vi "N-216 Stage Engine.vi"(0 "Unique Notifier Name":string, 11 "COM Port":string[](array[string])) -> ()   [LabVIEW 2016]
uses:
  Stages Controls/Stage Focus Control.ctl
  Stages Controls/Stage Status.ctl
  Stages Controls/Stage Actions.ctl
  Stages Controls/Stage Notifier Element.ctl
  PI GCS2 DLL/PI_GCS2_DLL_x64.dll
panel:
  in  "Reference":bool
  in  "Velocity (µm/s)":dbl=0.1 format="%#_13g"
  out "Number Connected":i32
  out "E-712 Found":bool
  in  "ReInitialize":bool
  in  "Abort":bool
  out "Status":T1
  in  "QUIT":bool
  in  "Focus Control":T2
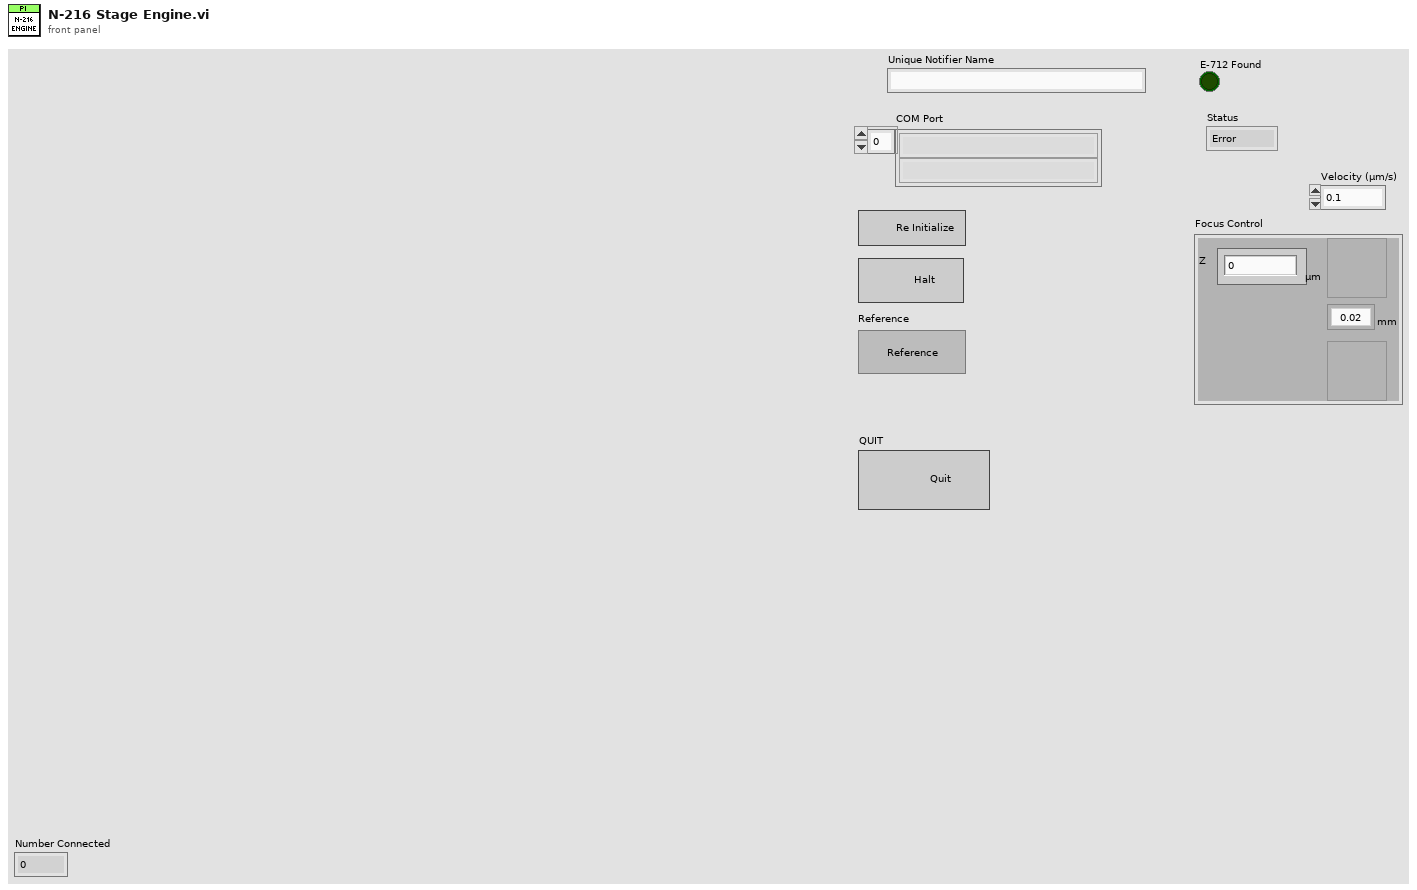
[diagram p1: front panel]
types:
  T1 = typedef "Stage Status.ctl" = enum16{"Error", "Abort", "Busy", "On Target"}
  T2 = typedef "Stage Focus Control.ctl" = cluster{"Focus Step (um)":enum16{"0.02", "0.05", "0.1", "0.5", "1", "2", "5", "10", "20"}, "Focus Up":bool, "Focus Down":bool, "Z ":dbl}
  T3 = typedef "Stage Notifier Element.ctl" = cluster{"Action":T4, "Axis":bool[], "Setpoint":dbl[], "Velocity":dbl, "Cmd Recvd?":bool, "Position":dbl[], "Status":T1, "Misc":variant}
  T4 = typedef "Stage Actions.ctl" = enum16{"Get Position", "MVR", "MOVE", "HALT", "ONTARGET", "ERROR", "REFERENCE", "INIT", "VELOCITY", "STATUS", "EXIT", "HOME", "ZEROPOS", "NANOPOS", "ANALOG", "QUIT"}
  T5 = enum32{"Invalid", "Standard", "Closed", "Hidden", "Minimized", "Maximized"}
  T6 = cluster{"Focus Step (um)":bool, "Focus Up":bool, "Focus Down":bool, "Z ":bool}
  T7 = enum16{"0.02", "0.05", "0.1", "0.5", "1", "2", "5", "10", "20"}
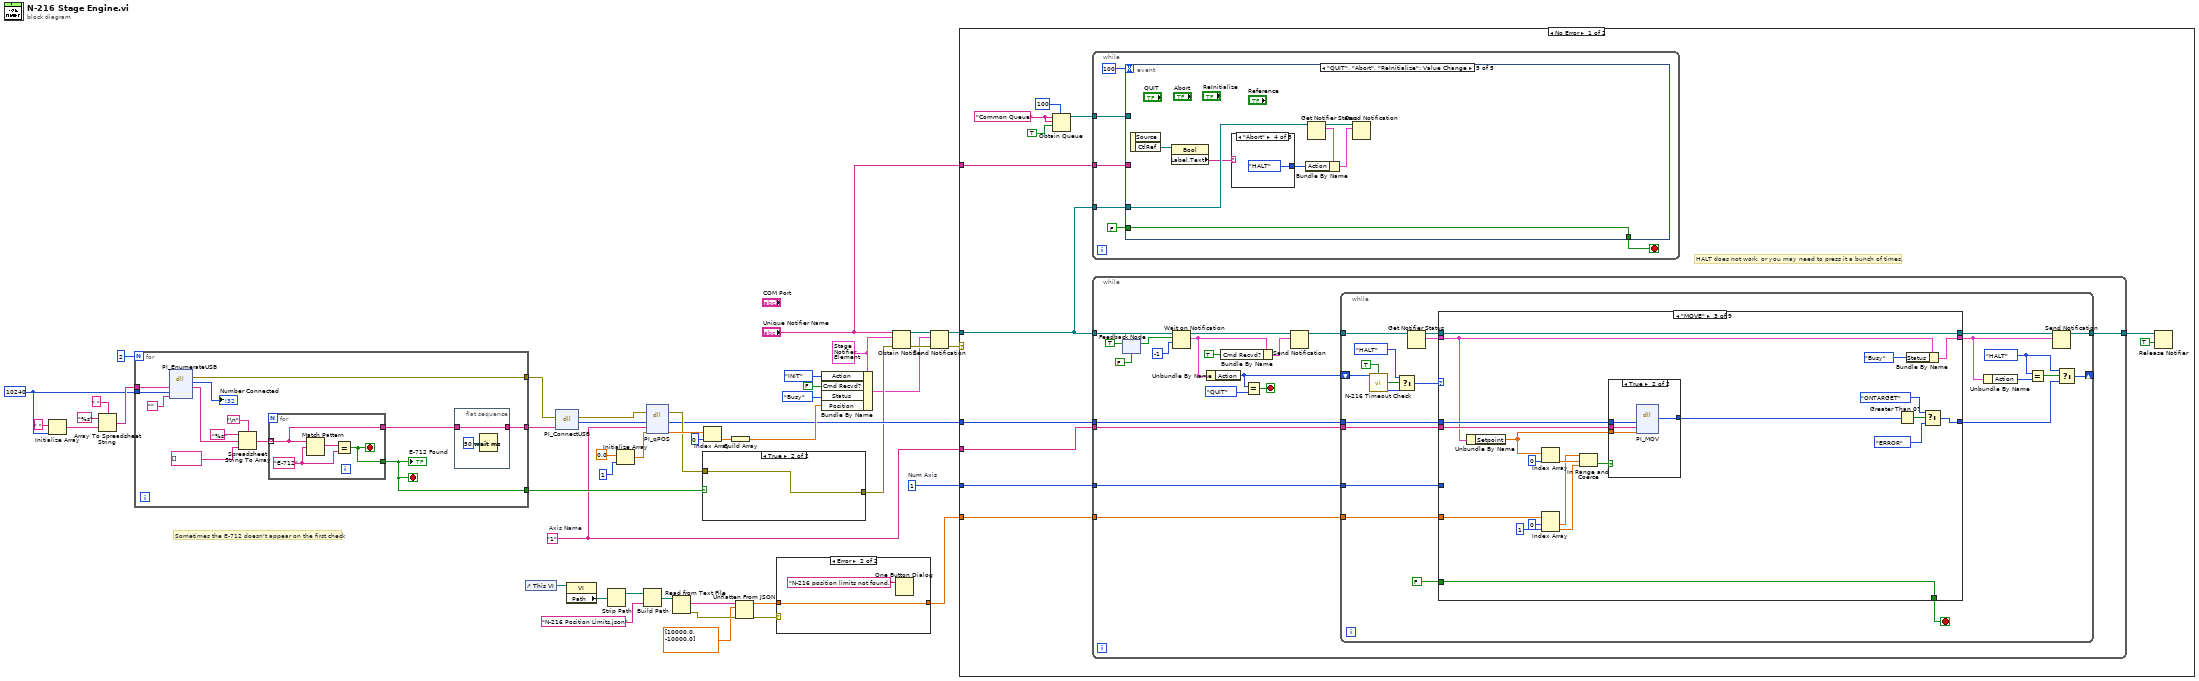
[diagram p0: block diagram]
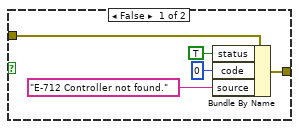
[diagram p3: hidden frame]
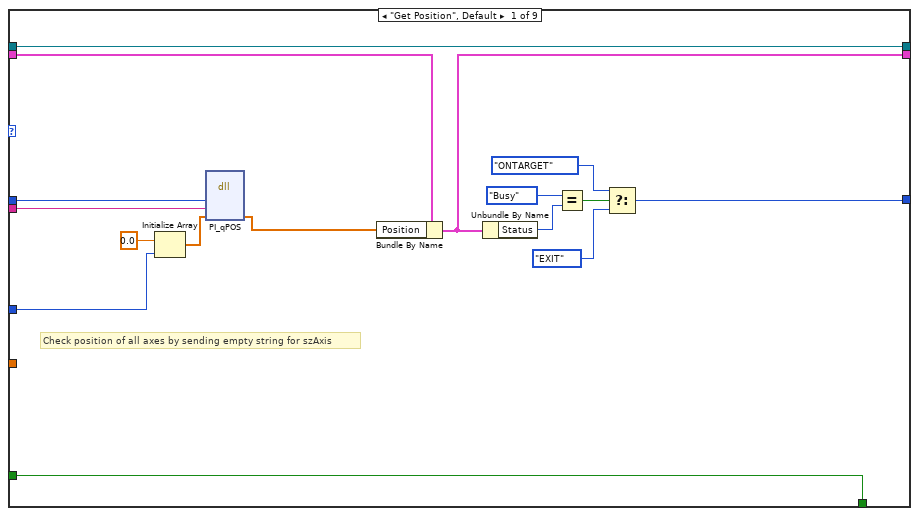
[diagram p4: hidden frame]
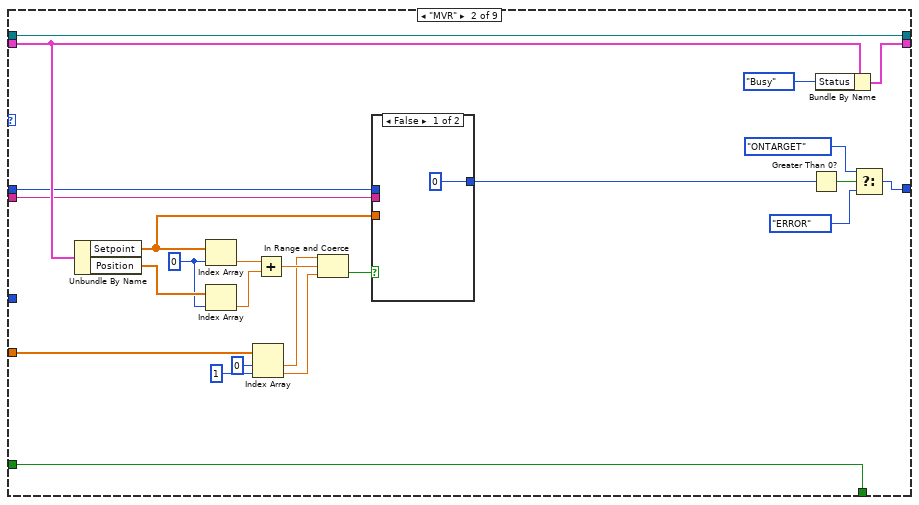
[diagram p5: hidden frame]
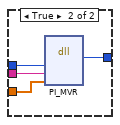
[diagram p6: hidden frame]
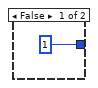
[diagram p7: hidden frame]
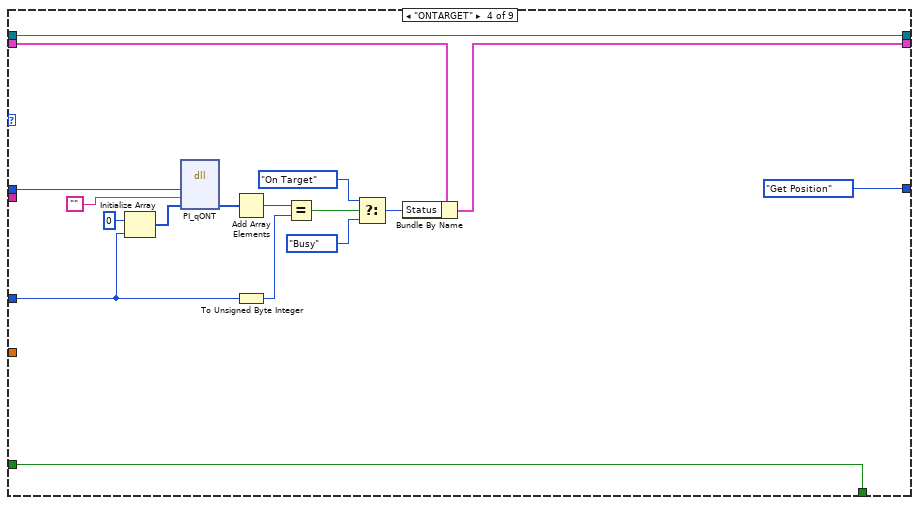
[diagram p8: hidden frame]
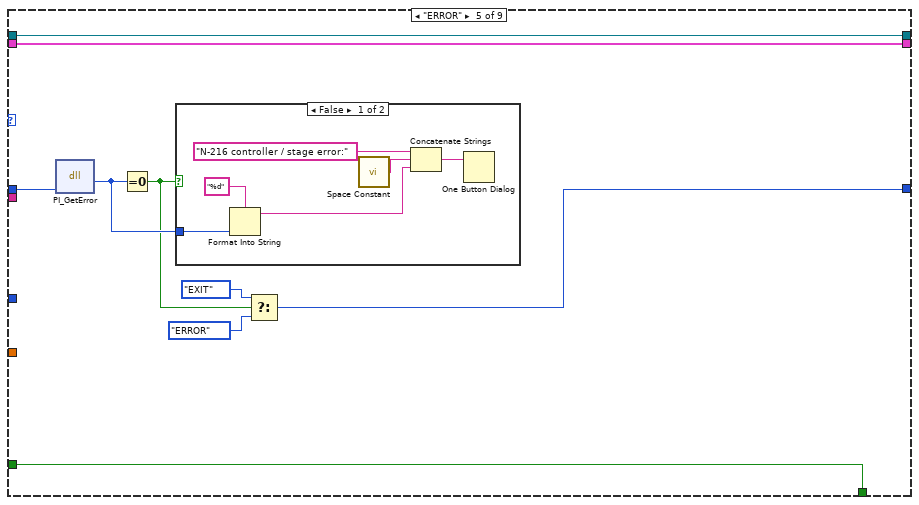
[diagram p9: hidden frame]
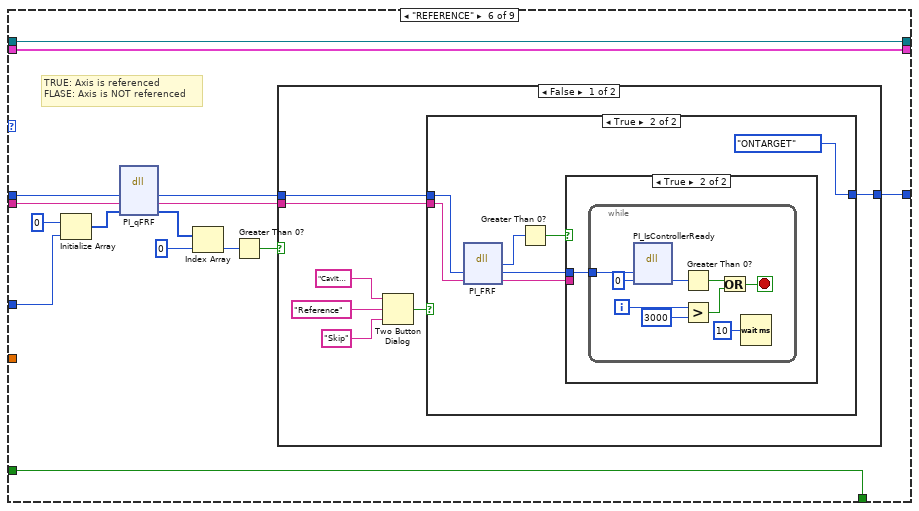
[diagram p11: hidden frame]
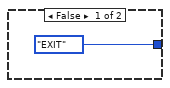
[diagram p12: hidden frame]
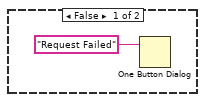
[diagram p13: hidden frame]
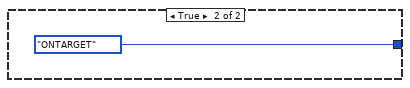
[diagram p14: hidden frame]
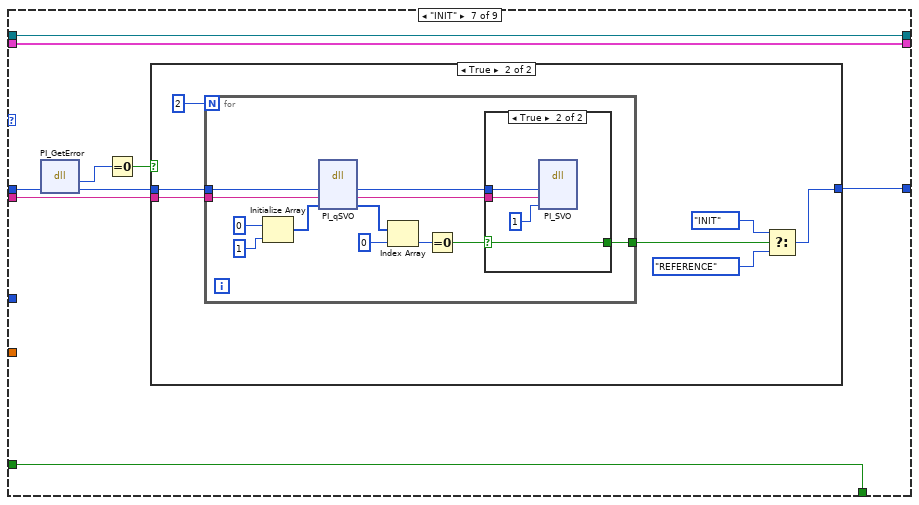
[diagram p15: hidden frame]
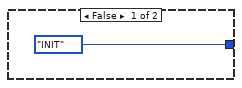
[diagram p16: hidden frame]
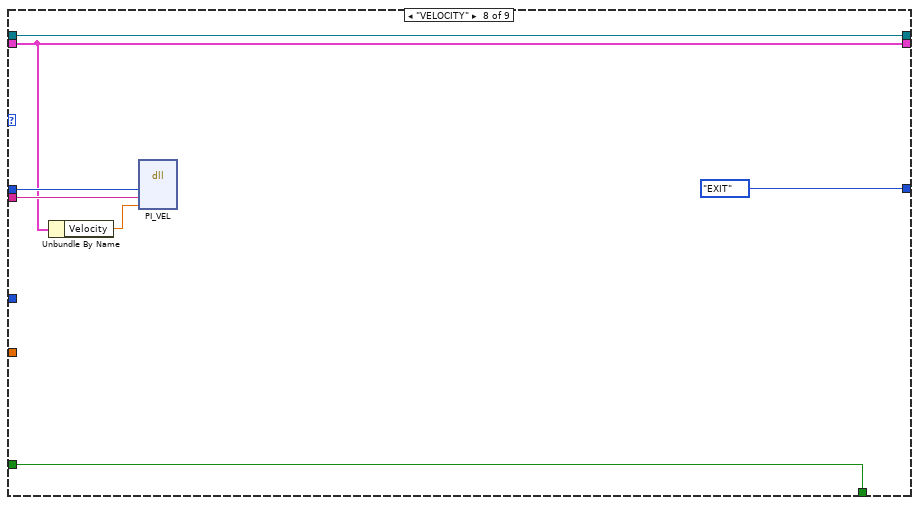
[diagram p18: hidden frame]
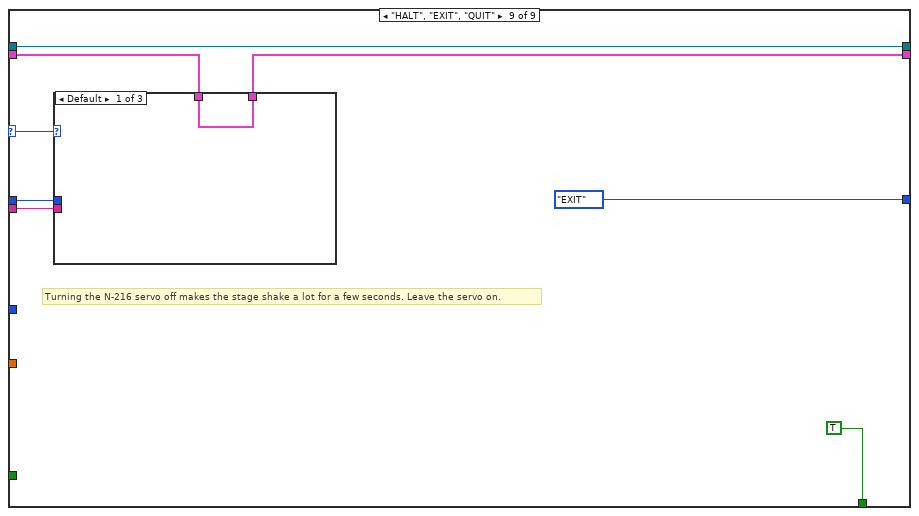
[diagram p19: hidden frame]
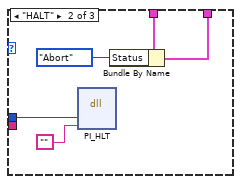
[diagram p20: hidden frame]
diagram:
  w13 = 1  # Num Axis
  w12 = "1"  # Axis Name
  w26 = T3 {"Action"=enum."Get Position", "Axis"=[], "Setpoint"=[], "Velocity"=0.5, "Cmd Recvd?"=FALSE, "Position"=[], "Status"=enum."Abort", "Misc"=variant} ("Stage Status")
  w40 = 10240 ("dimension size")
  # "Sometimes the E-712 doesn't appear on the first check"
  n1 = Initialize Array(" ", w40) -> (w44:string[])
  n2 = Array To Spreadsheet String(delimiter (Tab)=" ", array=w44, 3:"%s" ("format string")) -> (spreadsheet string=w41:string)
  n3 = for {
    N: 2 -> [_]
    tunnel: w41 -> [w53]
    tunnel: w40 -> [w52]
    tunnel: [w48] -> w38
    tunnel: [w47] -> w22
    tunnel: [w46] -> w32
    stop <- w47 stop-if-true
    n4 = dll-call lib="C:/Users/George Sirinakis/Documents/Microscope-Control/Device Library/Stages/PI/PI GCS2 DLL/PI_GCS2_DLL_x64.dll" fn="PI_EnumerateUSB"("szBuffer"=w53, "iBufferSize"=w52, "szFilter"="") -> (error out=w46:errorcluster, "return type"=→"Number Connected":i32, "szBuffer"=w50:string)  [unwired: 5 in, 1 out]
    n5 = Spreadsheet String To Array(delimiter (Tab)="\n", format string="%s", spreadsheet string=w50, array type (2D Dbl)=string[] []) -> (array=w55:string[])
    n6 = for {
      tunnel: w55 -> [w62] mode=indexing
      tunnel: [w62] -> w49
      tunnel: [w61] -> w47
      stop <- w61 stop-if-true
      w63 = "E-712"
      n7 = Match Pattern(string=w62, regular expression=w63) -> (match substring=w64:string)  [unwired: 1 in, 3 out]
      n8 = Equal?(x=w64, y=w63) -> (x = y?=w61:bool)
    }
    "E-712 Found" <- w47
    n9 = flat-sequence {
      tunnel: w49 -> [w60]
      tunnel: [w60] -> w48
      frame #0 {
        n10 = Wait (ms)(milliseconds to wait=u32 50) -> ()  [unwired: 1 out]
      }
    }
  }
  n11 = control-ref of="This VI"() -> (w11:refnum<vi>)
  n12 = dll-call lib="C:/Users/George Sirinakis/Documents/Microscope-Control/Device Library/Stages/PI/PI GCS2 DLL/PI_GCS2_DLL_x64.dll" fn="PI_ConnectUSB"(error in=w32, "szDescription"=w38) -> (error out=w33:errorcluster, "Device ID"=w34:i32)  [unwired: 3 in, 1 out]
  n13 = property class="VI"(reference=w11) -> ("Path"=w10:path)  [unwired: 1 in, 2 out]
  n14 = Strip Path(path=w10) -> (stripped path=w9:path)  [unwired: 1 out]
  n15 = Initialize Array(0.0 ("element"), 1 ("dimension size")) -> (w35:dbl[])
  n16 = Build Path(base path=w9, name or relative path="N-216 Position Limits.json") -> (appended path=w7:path)
  n17 = dll-call lib="C:/Users/George Sirinakis/Documents/Microscope-Control/Device Library/Stages/PI/PI GCS2 DLL/PI_GCS2_DLL_x64.dll" fn="PI_qPOS"(error in=w33, "Device ID"=w34, "szAxes"=w12, "pdValueArray"=w35) -> (error out=w21:errorcluster, "Device ID"=w20:i32, "pdValueArray"=w31:dbl[])  [unwired: 4 in, 1 out]
  n18 = Read from Text File(file (use dialog)=w7) -> (text=w6:string, error out=w5:errorcluster)  [unwired: 3 in, 2 out]
  n19 = case shown="True" w22 {
    tunnel: w21 -> [w69 w70]
    tunnel: [w67 w70] -> w19
    frame False {
      n20 = Bundle By Name(cluster=w69, "status"=TRUE, "code"=0, "source"="E-712 Controller not found.") -> (w67:errorcluster)
    }
    frame True {
    }
  }
  n21 = Index Array(array=w31, index=0) -> (element=w24:dbl)
  n22 = Build Array(w24) -> (w23:dbl[])
  n23 = Unflatten From JSON(JSON string=w6, type and defaults=dbl[] [10000.0, -10000.0], error in (no error)=w5) -> (value=w2:dbl[], error out=w3:errorcluster)  [unwired: 4 in]
  n24 = case shown="Error" w3 {
    tunnel: w2 -> [w71 w73]
    tunnel: [w71 w73] -> w1
    frame No Error {
    }
    frame Error {
      n25 = One Button Dialog(message="N-216 position limits not found.") -> ()  [unwired: 1 in, 1 out]
    }
  }
  n26 = Bundle By Name(cluster=w26, "Action"=Stage_Actions."INIT", "Cmd Recvd?"=FALSE, "Status"=Stage_Status."Busy", "Position"=w23) -> (w14:T3)
  n27 = Obtain Notifier(name (unnamed)="Unique Notifier Name", notification data type=w26, error in (no error)=w19) -> (notifier out=w18:refnum<notifier>, error out=w17:errorcluster)  [unwired: 1 in, 1 out]
  n28 = Send Notification(notification=w14, notifier=w18, error in (no error)=w17) -> (notifier out=w16:refnum<notifier>, error out=w15:errorcluster)
  n29 = case shown="No Error" w15 {
    selector: w15 -> [_ w427]
    tunnel: w16 -> [w79 w429]
    tunnel: "Unique Notifier Name" -> [w80 _]
    tunnel: w20 -> [w78 w428]
    tunnel: w12 -> [w77 _]
    tunnel: w13 -> [w75 _]
    tunnel: w1 -> [w74 _]
    frame No Error {
      w84 = "Common Queue" ("Unique Notifier Name")
      # "HALT does not work, or you may need to press it a bunch of times."
      n30 = Obtain Queue(max queue size (-1, unlimited)=100, name (unnamed)=w84, element data type=w84, create if not found? (T)=TRUE) -> (queue out=w81:refnum<queue>)  [unwired: 1 in, 2 out]
      n31 = while {
        tunnel: w79 -> [w339]
        tunnel: w81 -> [w338]
        tunnel: w80 -> [w337]
        stop <- w340 stop-if-true
        n32 = event shown="[4] \"QUIT\", \"Abort\", \"ReInitialize\": Value Change" {
          selector: _ -> [_ _ _ _ _]
          dyn-events: _ -> [_ _ _ _ _]
          timeout: 100 -> [_ _ _ _ _]
          tunnel: [w345 w358 w363 w412 w417] -> w340
          tunnel: w339 -> [w354 _ w368 w411 w420]
          tunnel: w338 -> [w347 _ _ _ _]
          tunnel: w337 -> [w342 _ _ _ _]
          tunnel: FALSE -> [_ w358 w363 w412 w417]
          event Timeout {
            n33 = event-data() -> ()  [unwired: 1 in, 1 out]
            n34 = call "Common Device Queue Get Command.vi"("Common Queue"=w347, "Notifier Name"=w342) -> ("Command"=w348:string)  [unwired: 12 in, 1 out]
            n35 = control-ref of="This VI"() -> (w349:refnum<vi>)
            n36 = call "Common Device Queue Execute Command.vi"("Common Command"=w348, "VI Refnum"=w349) -> ("Quit?"=w344:bool)  [unwired: 12 in, 1 out]
            n37 = Get Notifier Status(notifier=w354) -> (notifier out=w343:refnum<notifier>, current notification=w353:T3, error out=w351:errorcluster)  [unwired: 1 in, 2 out]
            n38 = Unbundle By Name(w353) -> ("Position"=w352:dbl[], "Status"=→"Status":T1)
            n39 = Unbundle By Name(w351) -> ("status"=w346:bool)
            n40 = Index Array(array=w352) -> (element=w355:dbl)  [unwired: 1 in]
            n41 = property on="Z" class="DigNum (strict)"("Value"=w355) -> ()  [unwired: 2 in, 2 out]
            n42 = Or(x=w344, y=w346) -> (x .or. y?=w345:bool)
            n43 = case shown="False" w344 {
              tunnel: w343 -> [_ w357]
              frame False {
              }
              frame True {
                n44 = Send Notification(notification=T3 {"Action"=enum."QUIT", "Axis"=[], "Setpoint"=[], "Velocity"=0.5, "Cmd Recvd?"=FALSE, "Position"=[], "Status"=enum."Error", "Misc"=variant} ("Stage Status"), notifier=w357) -> ()  [unwired: 1 in, 2 out]
              }
            }
          }
          event Application Instance Close? {
            n45 = event-data() -> ()  [unwired: 1 in, 5 out]
            n46 = control-ref of="This VI"() -> (w360:refnum<vi>)
            n47 = invoke class="VI" method="FP.Open"(reference=w360, "Activate"=TRUE ("Activate?"), "State"=T5."Standard") -> ()  [unwired: 2 in, 5 out]
            n48 = event-data("Discard?"=TRUE) -> ()  [unwired: 1 in, 1 out]
          }
          event Value Change {
            n49 = event-data() -> ("CtlRef"=w378:refnum<vi>, "OldVal"=w379:T2, "NewVal"=w372:T2)  [unwired: 1 in]
            n50 = Not Equal?(x=w379, y=w372) -> (x != y?=w377:T6)
            n51 = property class="Clust"(reference=w378) -> ("Controls[]"=w375:refnum<vi>[])  [unwired: 1 in, 2 out]
            n52 = Cluster To Array(cluster=w377) -> (array=w376:bool[])
            n53 = for {
              tunnel: w376 -> [w405] mode=indexing
              tunnel: [w404] -> w374
              tunnel: w375 -> [w404] mode=indexing
              stop <- w405 stop-if-true
            }
            n54 = property class="Ctl"(reference=w374) -> ("ClassName"=w373:string, "Label.Text"=w371:string)  [unwired: 1 in, 2 out]
            n55 = case shown="\"Boolean\"" w373 {
              tunnel: w372 -> [w387 w399 _]
              tunnel: w371 -> [w388 _ _]
              tunnel: [w382 w397 dbl[] []] -> w370
              tunnel: [w381 w396 w402] -> w369
              tunnel: [Stage_Actions."MVR" ("Action") Stage_Actions."MOVE" ("Action") Stage_Actions."Get Position" ("Action")] -> w367
              frame "Boolean" {
                n56 = Unbundle By Name(w387) -> ("Focus Step (um)"=w385:T7)
                n57 = Format Into String(w385) -> (resulting string=w386:string)  [unwired: 3 in, 1 out]
                n58 = Fract/Exp String To Number(string=w386) -> (number=w384:dbl)  [unwired: 3 in, 1 out]
                n59 = case shown="Default" w388 {
                  tunnel: w384 -> [w391 w392 w393]
                  tunnel: [w390 w392 w393] -> w383
                  frame "Focus Down" {
                    n60 = Negate(x=w391) -> (-x=w390:dbl)
                  }
                  frame "Focus Up" {
                  }
                  frame Default {
                  }
                }
                n61 = Build Array(w383) -> (w382:dbl[])
                n62 = Build Array(TRUE) -> (w381:bool[])
              }
              frame "Digital" {
                n63 = Unbundle By Name(w399) -> ("Z"=w398:dbl)
                n64 = Build Array(w398) -> (w397:dbl[])
                n65 = Build Array(TRUE) -> (w396:bool[])
              }
              frame Default {
                n66 = Build Array(FALSE) -> (w402:bool[])
              }
            }
            n67 = Get Notifier Status(notifier=w368) -> (notifier out=w366:refnum<notifier>, current notification=w365:T3)  [unwired: 1 in, 3 out]
            n68 = Bundle By Name(cluster=w365, "Action"=w367, "Setpoint"=w370, "Axis"=w369) -> (w364:T3)
            n69 = Send Notification(notification=w364, notifier=w366) -> ()  [unwired: 1 in, 2 out]
          }
          event "Velocity (µm/s)": Value Change {
            n70 = event-data() -> ("NewVal"=w408:dbl)  [unwired: 1 in]
            n71 = Get Notifier Status(notifier=w411) -> (notifier out=w407:refnum<notifier>, current notification=w410:T3)  [unwired: 1 in, 3 out]
            n72 = Bundle By Name(cluster=w410, "Action"=Stage_Actions."VELOCITY", "Velocity"=w408) -> (w406:T3)
            n73 = Send Notification(notification=w406, notifier=w407) -> ()  [unwired: 1 in, 2 out]
          }
          event "QUIT", "Abort", "ReInitialize": Value Change {
            n74 = event-data() -> ("CtlRef"=w419:refnum<vi>)  [unwired: 1 in, 1 out]
            n75 = property class="Bool"(reference=w419) -> ("Label.Text"=w418:string)  [unwired: 1 in, 2 out]
            n76 = case shown="\"Abort\"" w418 {
              tunnel: [Stage_Actions."EXIT" ("Action") Stage_Actions."QUIT" ("Action") Stage_Actions."INIT" ("Action") Stage_Actions."HALT" ("Action") Stage_Actions."REFERENCE" ("Action")] -> w416
              frame "Default", Default {
              }
              frame "QUIT" {
              }
              frame "ReInitialize" {
              }
              frame "Abort" {
              }
              frame "Reference" {
              }
            }
            n77 = Get Notifier Status(notifier=w420) -> (notifier out=w414:refnum<notifier>, current notification=w413:T3)  [unwired: 1 in, 3 out]
            n78 = Bundle By Name(cluster=w413, "Action"=w416) -> (w415:T3)
            n79 = Send Notification(notification=w415, notifier=w414) -> ()  [unwired: 1 in, 2 out]
          }
        }
      }
      n80 = while {
        tunnel: w79 -> [w100]
        tunnel: w78 -> [w98]
        tunnel: w77 -> [w97]
        tunnel: [w91] -> w76
        tunnel: w75 -> [w87]
        tunnel: w74 -> [w86]
        stop <- w103 stop-if-true
        n81 = feedback #1(FALSE) -> (w88:bool)
        n82 = feedback-in #1(TRUE) -> ()
        n83 = Wait on Notification(notifier=w100, ignore previous (F)=w88, timeout in ms (-1)=-1) -> (notifier out=w96:refnum<notifier>, notification=w94:T3)  [unwired: 1 in, 2 out]
        n84 = Unbundle By Name(w94) -> ("Action"=w99:T4)
        n85 = Bundle By Name(cluster=w94, "Cmd Recvd?"=TRUE) -> (w92:T3)
        n86 = Equal?(x=w99, y=Stage_Actions."QUIT") -> (x = y?=w103:bool)
        n87 = Send Notification(notification=w92, notifier=w96) -> (notifier out=w95:refnum<notifier>)  [unwired: 1 in, 1 out]
        n88 = while {
          tunnel: w98 -> [w124]
          tunnel: w95 -> [w114]
          shift-right: [w116] -> _
          shift-left: w99 -> [w109]
          tunnel: w97 -> [w123]
          tunnel: [w121] -> w91
          tunnel: w87 -> [w111]
          tunnel: w86 -> [w104]
          stop <- w125 stop-if-true
          w119 = Stage_Actions."HALT" ("Action")
          n89 = call "N-216 Timeout Check.vi"("Action"=w109, "User Input?"=TRUE) -> ("Timeout?"=w108:bool, "Action (Dup)"=w107:T4)  [unwired: 12 in]
          n90 = Select(t=Stage_Actions."HALT" ("y"), s=w108, f=w107) -> (s? t:f=w106:T4)
          n91 = Get Notifier Status(notifier=w114) -> (notifier out=w113:refnum<notifier>, current notification=w112:T3)  [unwired: 1 in, 3 out]
          n92 = case shown="\"MOVE\"" w106 {
            selector: w106 -> [_ _ _ _ _ _ _ _ w315]
            tunnel: w113 -> [w130 w165 w192 w214 w223 w244 w273 w312 w318]
            tunnel: FALSE -> [w139 w166 w191 w213 w221 w242 w278 w311 _]
            tunnel: [w139 w166 w191 w213 w221 w242 w278 w311 TRUE] -> w125
            tunnel: [w132 w161 w184 Stage_Actions."Get Position" ("y") w215 w234 w274 Stage_Actions."EXIT" ("y") Stage_Actions."EXIT" ("y")] -> w115
            tunnel: w124 -> [w140 w151 w190 w212 w220 w241 w280 w310 w317]
            tunnel: w123 -> [w127 w150 w189 _ _ w237 w275 w309 w316]
            tunnel: [w130 w165 w192 w214 w223 w244 w273 w312 w318] -> w122
            tunnel: [w138 w159 w183 w198 w222 w243 w272 w308 w313] -> w118
            tunnel: w112 -> [w131 w158 w181 w202 w222 w243 w272 w308 w314]
            tunnel: w111 -> [w129 _ _ w206 _ w230 _ _ _]
            tunnel: w104 -> [_ w147 w174 _ _ _ _ _ _]
            frame "Get Position", Default {
              # "Check position of all axes by sending empty string for szAxis"
              n93 = Initialize Array(0.0 ("element"), w129) -> (w142:dbl[])
              n94 = dll-call lib="C:/Users/George Sirinakis/Documents/Microscope-Control/Device Library/Stages/PI/PI GCS2 DLL/PI_GCS2_DLL_x64.dll" fn="PI_qPOS"("Device ID"=w140, "szAxes"=w127, "pdValueArray"=w142) -> ("pdValueArray"=w128:dbl[])  [unwired: 6 in, 2 out]
              n95 = Bundle By Name(cluster=w131, "Position"=w128) -> (w138:T3)
              n96 = Unbundle By Name(w138) -> ("Status"=w137:T1)
              n97 = Equal?(x=Stage_Status."Busy", y=w137) -> (x = y?=w135:bool)
              n98 = Select(t=Stage_Actions."ONTARGET" ("y"), s=w135, f=Stage_Actions."EXIT" ("y")) -> (s? t:f=w132:T4)
            }
            frame "MVR" {
              w156 = 0 ("index")
              n99 = Unbundle By Name(w158) -> ("Setpoint"=w149:dbl[], "Position"=w157:dbl[])
              n100 = Index Array(array=w149, index=w156) -> (element=w155:dbl)
              n101 = Index Array(array=w157, index=w156) -> (element=w154:dbl)
              n102 = Index Array(array=w147, index #1=0 ("index"), index #2=1 ("index")) -> (element #1=w144:dbl, element #2=w143:dbl)
              n103 = Add(x=w155, y=w154) -> (x+y=w153:dbl)
              n104 = In Range and Coerce(upper limit=w144, x=w153, lower limit=w143) -> (In Range?=w152:bool)  [unwired: 1 out]
              n105 = case shown="False" w152 {
                tunnel: w151 -> [_ w171]
                tunnel: w150 -> [_ w170]
                tunnel: w149 -> [_ w169]
                tunnel: [u8 0 ("Success") w168] -> w148
                frame False {
                }
                frame True {
                  n106 = dll-call lib="C:/Users/George Sirinakis/Documents/Microscope-Control/Device Library/Stages/PI/PI GCS2 DLL/PI_GCS2_DLL_x64.dll" fn="PI_MVR"("Device ID"=w171, "szAxes"=w170, "pdValueArray"=w169) -> ("Success"=w168:u8)  [unwired: 6 in, 2 out]
                }
              }
              n107 = Greater Than 0?(x=w148) -> (x > 0?=w164:bool)
              n108 = Bundle By Name(cluster=w158, "Status"=Stage_Status."Busy") -> (w159:T3)
              n109 = Select(t=Stage_Actions."ONTARGET" ("Action"), s=w164, f=Stage_Actions."ERROR" ("Action")) -> (s? t:f=w161:T4)
            }
            frame "MOVE" {
              n110 = Unbundle By Name(w181) -> ("Setpoint"=w180:dbl[])
              n111 = Index Array(array=w180, index=0) -> (element=w178:dbl)
              n112 = Index Array(array=w174, index #1=0 ("index"), index #2=1 ("index")) -> (element #1=w173:dbl, element #2=w172:dbl)
              n113 = In Range and Coerce(upper limit=w173, x=w178, lower limit=w172) -> (In Range?=w177:bool)  [unwired: 1 out]
              n114 = case shown="True" w177 {
                tunnel: w190 -> [_ w197]
                tunnel: w189 -> [_ w196]
                tunnel: [u8 1 ("Success") w195] -> w188
                tunnel: w180 -> [_ w194]
                frame False {
                }
                frame True {
                  n115 = dll-call lib="C:/Users/George Sirinakis/Documents/Microscope-Control/Device Library/Stages/PI/PI GCS2 DLL/PI_GCS2_DLL_x64.dll" fn="PI_MOV"("Device ID"=w197, "szAxes"=w196, "pdValueArray"=w194) -> ("Success"=w195:u8)  [unwired: 6 in, 2 out]
                }
              }
              n116 = Greater Than 0?(x=w188) -> (x > 0?=w187:bool)
              n117 = Bundle By Name(cluster=w181, "Status"=Stage_Status."Busy") -> (w183:T3)
              n118 = Select(t=Stage_Actions."ONTARGET" ("Action"), s=w187, f=Stage_Actions."ERROR" ("Action")) -> (s? t:f=w184:T4)
            }
            frame "ONTARGET" {
              n119 = Initialize Array(u8 0 ("element"), w206) -> (w210:u8[])
              n120 = dll-call lib="C:/Users/George Sirinakis/Documents/Microscope-Control/Device Library/Stages/PI/PI GCS2 DLL/PI_GCS2_DLL_x64.dll" fn="PI_qONT"("Device ID"=w212, "szAxes"="", "pdValueArray"=w210) -> ("pdValueArray"=w208:u8[])  [unwired: 6 in, 2 out]
              n121 = Add Array Elements(numeric array=w208) -> (sum=w207:u8)
              n122 = To Unsigned Byte Integer(number=w206) -> (unsigned 8bit integer=w205:u8)
              n123 = Equal?(x=w207, y=w205) -> (x = y?=w204:bool)
              n124 = Select(t=Stage_Status."On Target" ("Status"), s=w204, f=Stage_Status."Busy" ("Status")) -> (s? t:f=w199:T1)
              n125 = Bundle By Name(cluster=w202, "Status"=w199) -> (w198:T3)
            }
            frame "ERROR" {
              n126 = dll-call lib="C:/Users/George Sirinakis/Documents/Microscope-Control/Device Library/Stages/PI/PI GCS2 DLL/PI_GCS2_DLL_x64.dll" fn="PI_GetError"("Device ID"=w220) -> ("Error Code"=w219:i32)  [unwired: 4 in, 2 out]
              n127 = Equal To 0?(x=w219) -> (x = 0?=w218:bool)
              n128 = case shown="False" w218 {
                tunnel: w219 -> [w227 _]
                frame False {
                  n129 = Format Into String(format string="%d", w227) -> (resulting string=w225:string)  [unwired: 2 in, 1 out]
                  n130 = call <vilib>:"Space Constant.vi"() -> ("String"=w228:string)
                  n131 = Concatenate Strings("N-216 controller / stage error:", w228, w225) -> (w224:string)
                  n132 = One Button Dialog(message=w224) -> ()  [unwired: 1 in, 1 out]
                }
                frame True {
                }
              }
              n133 = Select(t=Stage_Actions."EXIT", s=w218, f=Stage_Actions."ERROR" ("Action")) -> (s? t:f=w215:T4)
            }
            frame "REFERENCE" {
              # "TRUE: Axis is referenced\nFLASE: Axis is NOT referenced"
              n134 = Initialize Array(u8 0 ("element"), w230) -> (w239:u8[])
              n135 = dll-call lib="C:/Users/George Sirinakis/Documents/Microscope-Control/Device Library/Stages/PI/PI GCS2 DLL/PI_GCS2_DLL_x64.dll" fn="PI_qFRF"("Device ID"=w241, "szAxes"=w237, "pdValueArray"=w239) -> ("Device ID"=w232:i32, "szAxes"=w233:string, "pdValueArray"=w238:u8[])  [unwired: 4 in, 2 out]
              n136 = Index Array(array=w238, index=0) -> (element=w235:u8)
              n137 = Greater Than 0?(x=w235) -> (x > 0?=w231:bool)
              n138 = case shown="False" w231 {
                tunnel: [w245 Stage_Actions."ONTARGET" ("Action")] -> w234
                tunnel: w233 -> [w246 _]
                tunnel: w232 -> [w247 _]
                frame False {
                  n139 = Two Button Dialog(message="Cavity stage (N-216) is not referenced.", 1:"Skip" ("F button name (\"Cancel\")"), 2:"Reference" ("T button name (\"OK\")")) -> (T button?=w248:bool)
                  n140 = case shown="True" w248 {
                    tunnel: w247 -> [_ w253]
                    tunnel: w246 -> [_ w254]
                    tunnel: [Stage_Actions."EXIT" ("Action") Stage_Actions."ONTARGET" ("Action")] -> w245
                    frame False {
                    }
                    frame True {
                      n141 = dll-call lib="C:/Users/George Sirinakis/Documents/Microscope-Control/Device Library/Stages/PI/PI GCS2 DLL/PI_GCS2_DLL_x64.dll" fn="PI_FRF"("Device ID"=w253, "szAxes"=w254) -> ("Success"=w255:u8, "Device ID"=w257:i32, "szAxes"=w258:string)  [unwired: 3 in, 2 out]
                      n142 = Greater Than 0?(x=w255) -> (x > 0?=w256:bool)
                      n143 = case shown="True" w256 {
                        tunnel: w257 -> [_ w261]
                        tunnel: w258 -> [_ _]
                        frame False {
                          n144 = One Button Dialog(message="Request Failed") -> ()  [unwired: 1 in, 1 out]
                        }
                        frame True {
                          n145 = while {
                            tunnel: w261 -> [w270]
                            i -> [w268]
                            stop <- w263 stop-if-true
                            n146 = dll-call lib="C:/Users/George Sirinakis/Documents/Microscope-Control/Device Library/Stages/PI/PI GCS2 DLL/PI_GCS2_DLL_x64.dll" fn="PI_IsControllerReady"("Device ID"=w270, "piControllerReady"=0) -> ("piControllerReady"=w266:i32)  [unwired: 5 in, 2 out]
                            n147 = Greater Than 0?(x=w266) -> (x > 0?=w265:bool)
                            n148 = Greater?(x=w268, y=3000) -> (0:w264:bool)
                            n149 = Or(x=w265, y=w264) -> (x .or. y?=w263:bool)
                            n150 = Wait (ms)(milliseconds to wait=u32 10) -> ()  [unwired: 1 out]
                          }
                        }
                      }
                    }
                  }
                }
                frame True {
                }
              }
            }
            frame "INIT" {
              n151 = dll-call lib="C:/Users/George Sirinakis/Documents/Microscope-Control/Device Library/Stages/PI/PI GCS2 DLL/PI_GCS2_DLL_x64.dll" fn="PI_GetError"("Device ID"=w280) -> ("Error Code"=w279:i32, "Device ID"=w276:i32)  [unwired: 3 in, 2 out]
              n152 = Equal To 0?(x=w279) -> (x = 0?=w277:bool)
              n153 = case shown="True" w277 {
                tunnel: w276 -> [_ w288]
                tunnel: w275 -> [_ w287]
                tunnel: [Stage_Actions."INIT" ("Action") w284] -> w274
                frame False {
                }
                frame True {
                  n154 = for {
                    N: 2 -> [_]
                    tunnel: w288 -> [w297]
                    tunnel: w287 -> [w296]
                    tunnel: [w289] -> w285
                    n155 = Initialize Array(u8 0 ("element"), 1 ("dimension size")) -> (w300:u8[])
                    n156 = dll-call lib="C:/Users/George Sirinakis/Documents/Microscope-Control/Device Library/Stages/PI/PI GCS2 DLL/PI_GCS2_DLL_x64.dll" fn="PI_qSVO"("Device ID"=w297, "szAxes"=w296, "pdValueArray"=w300) -> ("Device ID"=w290:i32, "szAxes"=w291:string, "pdValueArray"=w295:u8[])  [unwired: 4 in, 2 out]
                    n157 = Index Array(array=w295, index=0) -> (element=w293:u8)
                    n158 = Equal To 0?(x=w293) -> (x = 0?=w292:bool)
                    n159 = case shown="True" w292 {
                      selector: w292 -> [w301 w302]
                      tunnel: w291 -> [_ w304]
                      tunnel: w290 -> [_ w305]
                      tunnel: [w301 w302] -> w289
                      frame False {
                      }
                      frame True {
                        n160 = dll-call lib="C:/Users/George Sirinakis/Documents/Microscope-Control/Device Library/Stages/PI/PI GCS2 DLL/PI_GCS2_DLL_x64.dll" fn="PI_SVO"("Device ID"=w305, "szAxes"=w304, "pdValueArray"=u8 1) -> ()  [unwired: 7 in, 2 out]
                      }
                    }
                  }
                  n161 = Select(t=Stage_Actions."INIT" ("Action"), s=w285, f=Stage_Actions."REFERENCE" ("Action")) -> (s? t:f=w284:T4)
                }
              }
            }
            frame "VELOCITY" {
              n162 = Unbundle By Name(w308) -> ("Velocity"=w307:dbl)
              n163 = dll-call lib="C:/Users/George Sirinakis/Documents/Microscope-Control/Device Library/Stages/PI/PI GCS2 DLL/PI_GCS2_DLL_x64.dll" fn="PI_VEL"("Device ID"=w310, "szAxes"=w309, "pdValueArray"=w307) -> ()  [unwired: 7 in, 2 out]
            }
            frame "HALT", "EXIT", "QUIT" {
              # "Turning the N-216 servo off makes the stage shake a lot for a few seconds. Leave the servo on."
              n164 = case shown="Default" w315 {
                tunnel: w317 -> [_ w326 w330]
                tunnel: w316 -> [_ _ w329]
                tunnel: w314 -> [w321 w324 w327]
                tunnel: [w321 w322 w327] -> w313
                frame Default {
                }
                frame "HALT" {
                  n165 = dll-call lib="C:/Users/George Sirinakis/Documents/Microscope-Control/Device Library/Stages/PI/PI GCS2 DLL/PI_GCS2_DLL_x64.dll" fn="PI_HLT"("Device ID"=w326, "szAxes"="") -> ()  [unwired: 6 in, 2 out]
                  n166 = Bundle By Name(cluster=w324, "Status"=Stage_Status."Abort") -> (w322:T3)
                }
                frame "QUIT" {
                  n167 = disable-structure shown="Disabled" {
                    disable-tunnel: w330 -> [w333 w335]
                    disable-tunnel: w329 -> [w332 _]
                    disable-tunnel: [w331 w335] -> w328
                    frame Disabled {
                      n168 = dll-call lib="C:/Users/George Sirinakis/Documents/Microscope-Control/Device Library/Stages/PI/PI GCS2 DLL/PI_GCS2_DLL_x64.dll" fn="PI_SVO"("Device ID"=w333, "szAxes"=w332, "pdValueArray"=u8 0) -> ("Device ID"=w331:i32)  [unwired: 6 in, 2 out]
                    }
                    frame Enabled {
                    }
                  }
                  n169 = dll-call lib="C:/Users/George Sirinakis/Documents/Microscope-Control/Device Library/Stages/PI/PI GCS2 DLL/PI_GCS2_DLL_x64.dll" fn="PI_CloseConnection"("Device ID"=w328) -> ()  [unwired: 5 in, 2 out]
                }
              }
            }
          }
          n170 = Unbundle By Name(w118) -> ("Action"=w117:T4)
          n171 = Equal?(x=w119, y=w117) -> (x = y?=w120:bool)
          n172 = Send Notification(notification=w118, notifier=w122) -> (notifier out=w121:refnum<notifier>)  [unwired: 1 in, 1 out]
          n173 = Select(t=w119, s=w120, f=w115) -> (s? t:f=w116:T4)
        }
      }
      n174 = Release Notifier(notifier=w76, force destroy? (F)=TRUE) -> ()  [unwired: 1 in, 3 out]
    }
    frame Error {
      n175 = dll-call lib="C:/Users/George Sirinakis/Documents/Microscope-Control/Device Library/Stages/PI/PI GCS2 DLL/PI_GCS2_DLL_x64.dll" fn="PI_CloseConnection"(error in=w427, "Device ID"=w428) -> (error out=w426:errorcluster)  [unwired: 4 in, 1 out]
      n176 = Release Notifier(notifier=w429, force destroy? (F)=TRUE, error in (no error)=w426) -> (error out=w434:errorcluster)  [unwired: 2 out]
      n177 = Unbundle By Name(w434) -> ("source"=w431:string)
      n178 = Concatenate Strings("N-216 Initialization Error", "\r", w431) -> (w430:string)
      n179 = One Button Dialog(message=w430) -> ()  [unwired: 1 in, 1 out]
    }
  }
